vi "pm1-mcu.vi"() -> ()   [LabVIEW 2015]
uses:
  <vilib>/myRIO/Common/Instrument Driver Framework/myRIO v1.0/UART/vis/myRIO v1.0 Close UART.vi
  <vilib>/FPGAPlugInAG/myRIO-1900/niLvFpga_Open_myRIO-1900.vi
  <vilib>/rvi/interface/common/dynamic/niFpgaDynamicAddResources.vi
  <vilib>/imath/engines/lvmath2/RunTimeEngine/BuiltInFunctions/fix/NIMS_fix(DBL-S).vi
  <vilib>/imath/engines/lvmath2/RunTimeEngine/BuiltInFunctions/rand/NIMS_rand().vi
  <vilib>/imath/engines/lvmath2/RunTimeEngine/ErrorHandling/NIMS_Error From Error Code.vi
  <vilib>/imath/engines/lvmath2/RunTimeEngine/NodeEndStatement/NIMS_NodeEndStatement_Output.vi
  <instcachedir>/0/NIMS_NodeEndStatement_Output_53EC0D466D134D7ABD903AC30B43404B.lvgen/NIMS_NodeEndStatement_Output_53EC0D466D134D7ABD903AC30B43404B_010.vi
  <instcachedir>/0/NIMS_NodeEndStatement_Output_53EC0D466D134D7ABD903AC30B43404B.lvgen/NIMS_NodeEndStatement_Output_53EC0D466D134D7ABD903AC30B43404B_001.vi
  <vilib>/imath/engines/lvmath2/RunTimeEngine/ErrorHandling/NIMS_Finalize Error.vi
  <vilib>/Utility/error.llb/Error Cluster From Error Code.vi
  <vilib>/rvi/errors/niLvFpgaAdjustHostInterfaceError.vi
  <vilib>/FPGAPlugInAG/Dynamic/niLvFpga_Close_Dynamic.vi
  <vilib>/myRIO/Common/Instrument Driver Framework/Utilities/vis/FPGA Ref Manager.vi
  <vilib>/myRIO/Common/Instrument Driver Framework/myRIO v1.0/myRIO v1.0 Reset FPGA.vi
  <vilib>/myRIO/Common/Instrument Driver Framework/myRIO v1.0/IRQ/vis/myRIO v1.0 IRQ Info FGV.vi
  <vilib>/myRIO/Common/Instrument Driver Framework/myRIO v1.0/IRQ/vis/myRIO v1.0 Timer IRQ Info FGV.vi
  <vilib>/myRIO/Common/Instrument Driver Framework/myRIO v1.0/IRQ/vis/myRIO v1.0 ISR Agent.vi
  <vilib>/rvi/interface/nirviOpenFPGA/nirviOpenFPGA.xnode
  FPGA Bitfiles/pm1_FPGATarget_pm1-fpga_HhK76n5Wd-Q.lvbitx
  pm1-fpga.vi
  <vilib>/rvi/interface/nirviReadWriteControl/nirviReadWriteControl.xnode
  <vilib>/rvi/interface/nirviCloseFPGA/nirviCloseFPGA.xnode
  <vilib>/myRIO/Instrument Drivers/Utilities/Utilities.lvlib
  NiFpgaLv.dll
  <vilib>/rvi/interface/Simulation/niFpgaSimulationCallBeginRW.vi
panel:
  in  "Time Between Note Change (mSec)":i32
  in  "Test Button Three":bool
  in  "Test Button Two":bool
  in  "Test Button One":bool
  in  "Randomize Inputs for Training Data Input":bool
  out "Number of Buttons Being Pressed":dbl format="%#_13g"
  out "Interval Between Consecutive Notes":dbl format="%#_13g"
  out "Note 6":string
  out "Note 5":string
  out "Note 4":string
  out "Note 3":string
  out "Note 2":string
  out "Note 1":string
  out "Octave6":dbl format="%#_13g"
  out "Octave5":dbl format="%#_13g"
  out "Octave4":dbl format="%#_13g"
  out "Octave3":dbl format="%#_13g"
  out "Octave2":dbl format="%#_13g"
  out "Octave1":dbl format="%#_13g"
  out "Button6":bool
  out "Button5":bool
  out "Button4":bool
  out "Button3":bool
  out "Button2":bool
  out "Button1":bool
  out "Waveform Chart":sgl(graph)
  out "Octave":dbl format="%#_13g"
  out "pitch":dbl format="%#_13g"
  in  "Volume":dbl(slide) scale=0.0..10.0
  out "frequency 6":dbl format="%#_13g"
  out "frequency 5":dbl format="%#_13g"
  out "frequency 4":dbl format="%#_13g"
  out "frequency 3":dbl format="%#_13g"
  out "frequency 2":dbl format="%#_13g"
  out "frequency 1":dbl format="%#_13g"
  out "error out":errorcluster
  in  "stop":bool
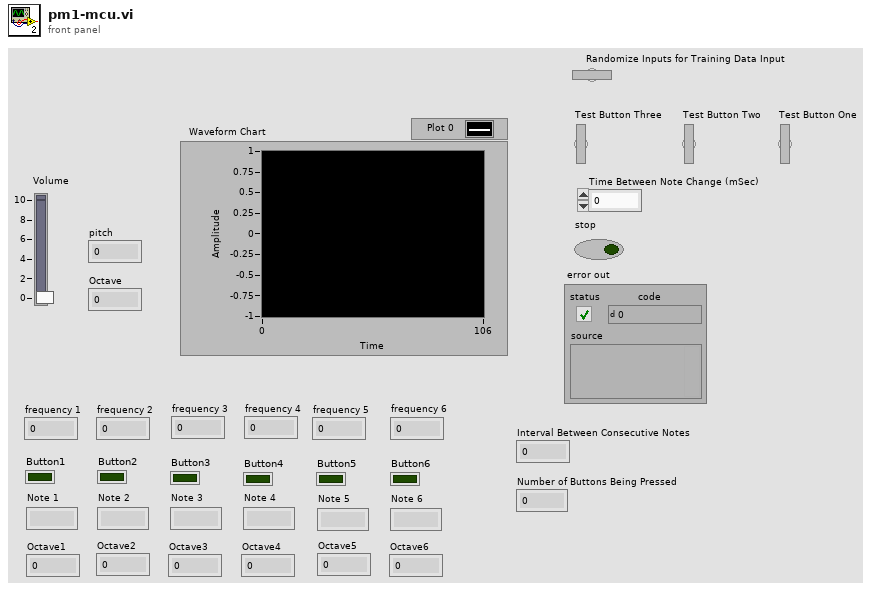
[diagram p1: front panel]
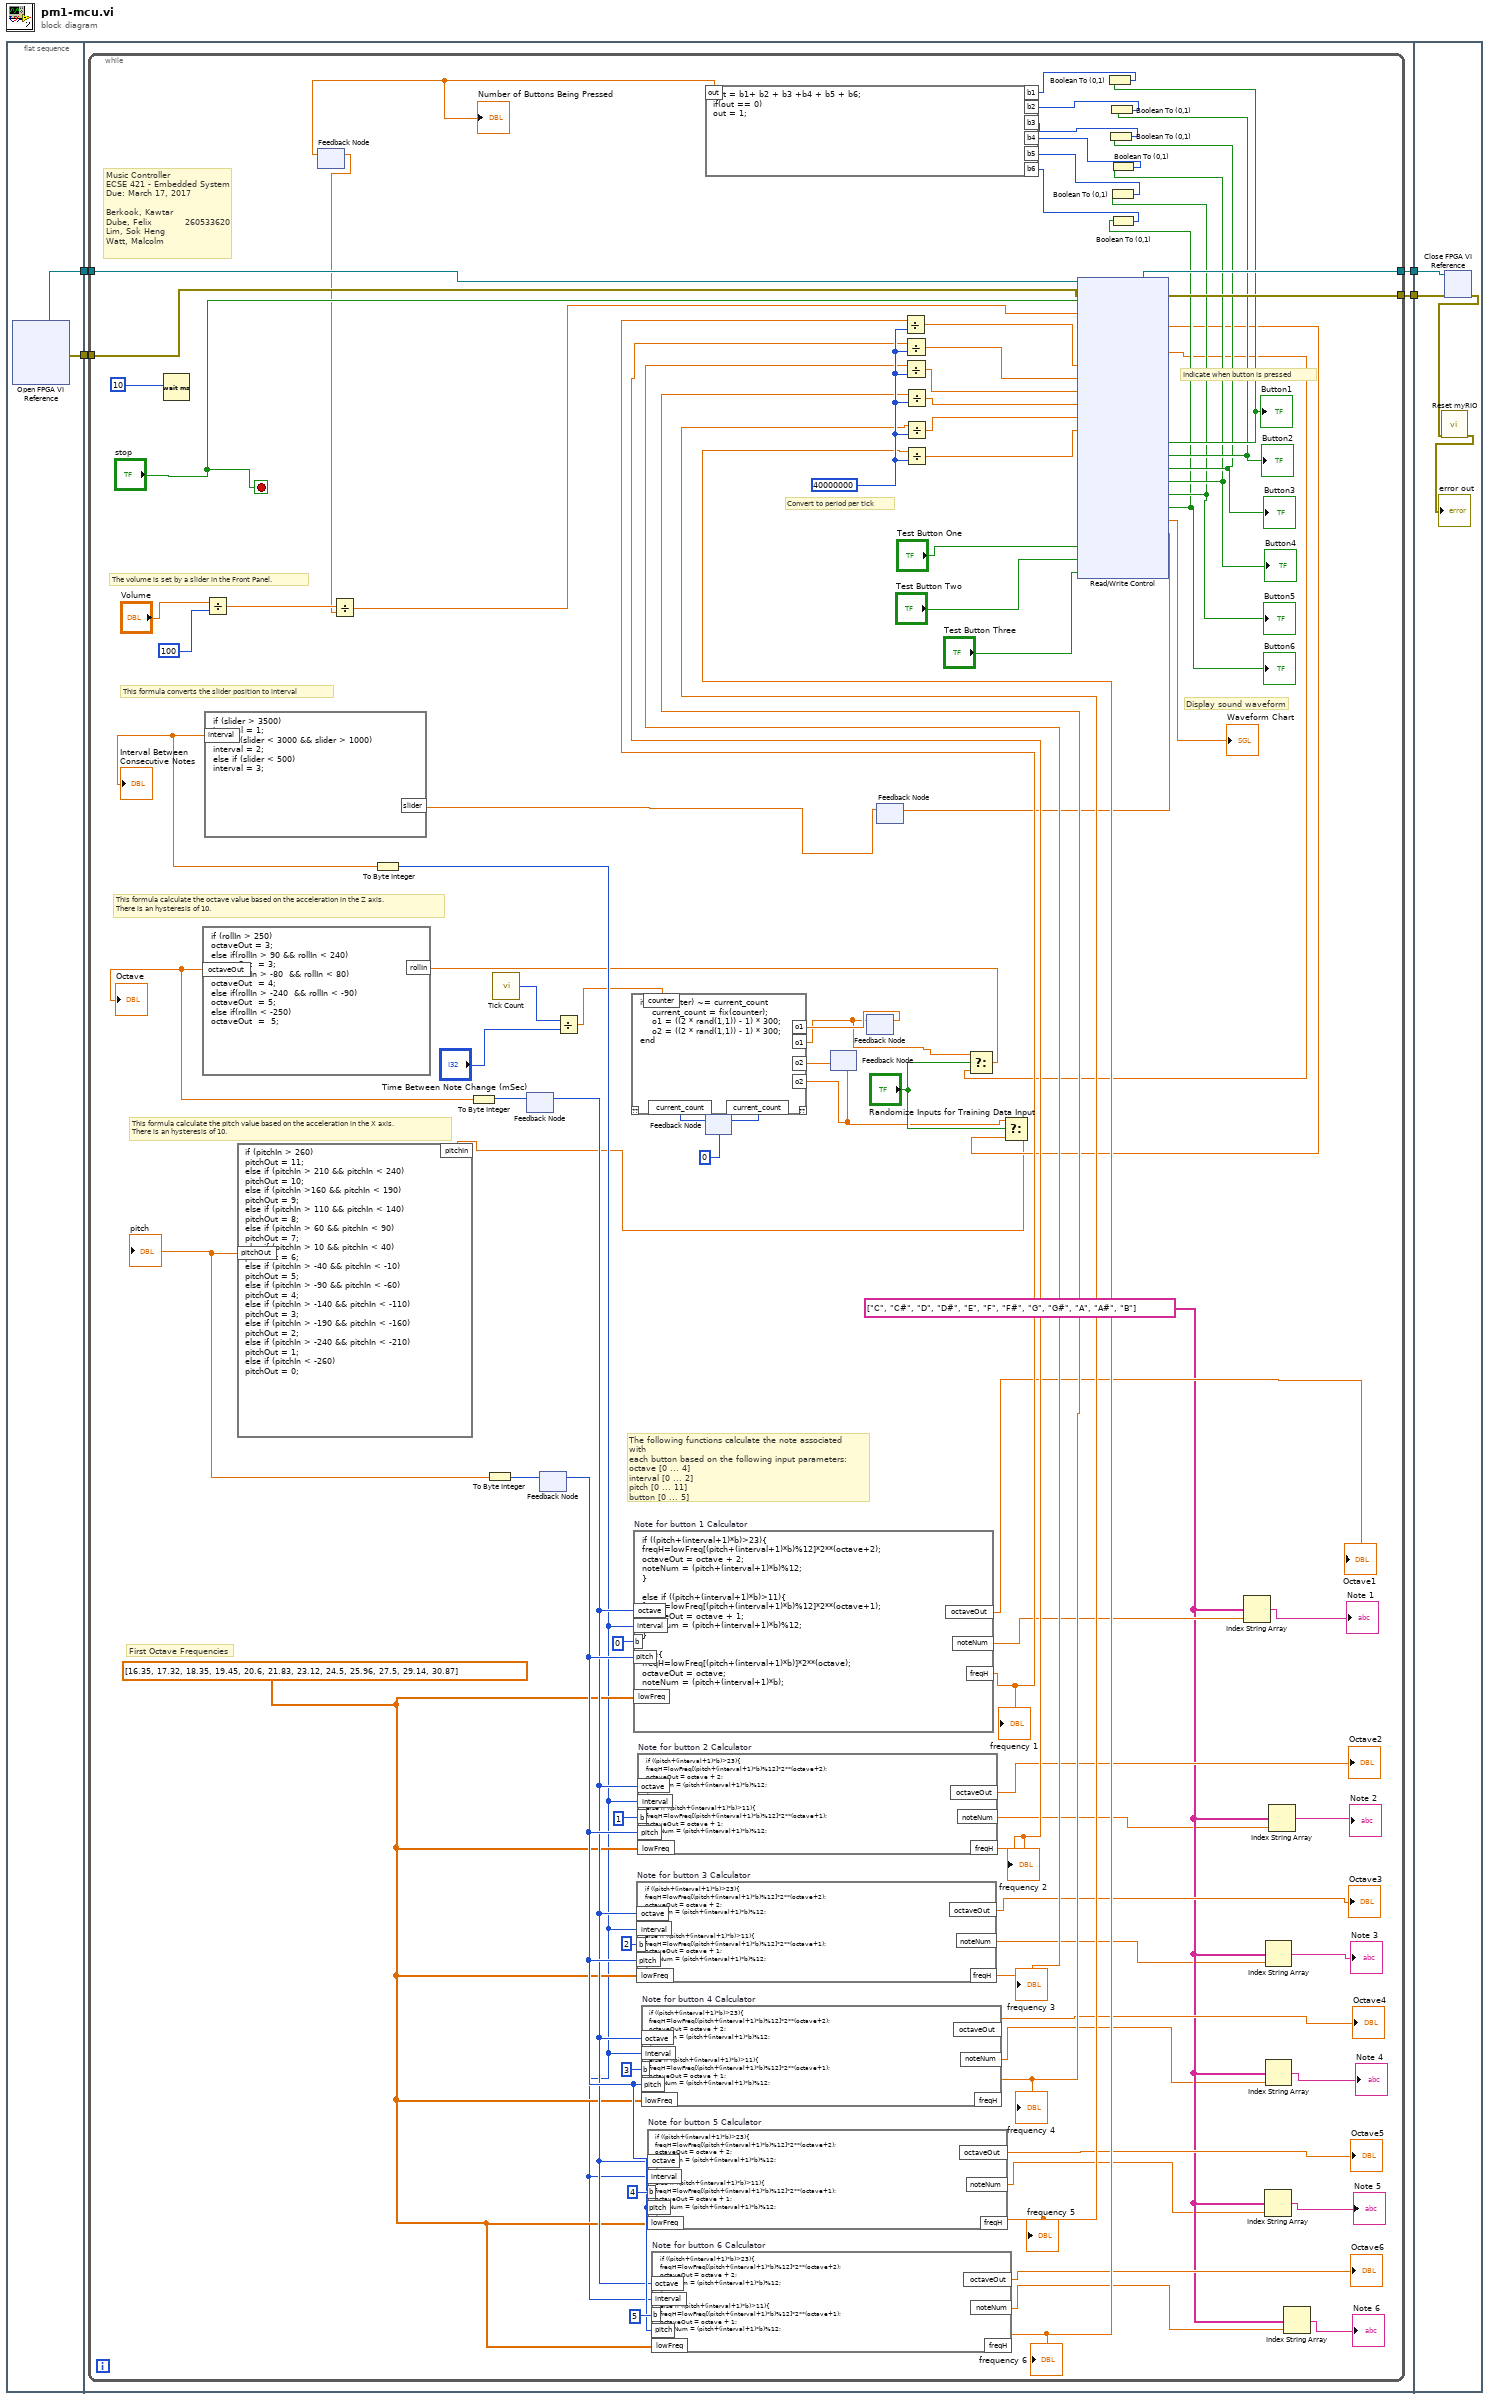
[diagram p0: block diagram]
diagram:
  n1 = flat-sequence {
    tunnel: [w6] -> w4
    tunnel: [w5] -> w2
    tunnel: w4 -> [w10]
    tunnel: [w9] -> w3
    tunnel: w2 -> [w8]
    tunnel: [w7] -> w1
    tunnel: w3 -> [w202]
    tunnel: w1 -> [w201]
    frame #0 {
      n2 = xnode "Open FPGA VI Reference"() -> ("FPGA VI Reference Out"=w6:refnum<k20>, "error out"=w5:errorcluster)  [unwired: 2 in]
    }
    frame #1 {
      n3 = while {
        tunnel: w10 -> [w102]
        tunnel: [w101] -> w9
        tunnel: w8 -> [w99]
        tunnel: [w98] -> w7
        stop <- "stop" stop-if-true
        w60 = string[] ["C", "C#", "D", "D#", "E", "F", "F#", "G", "G#", "A", "A#", "B"]
        w72 = dbl[] [16.35, 17.32, 18.35, 19.45, 20.6, 21.83, 23.12, 24.5, 25.96, 27.5, 29.14, 30.87] ("Low Frequency (Hz) 2")
        w85 = 40000000
        # "This formula converts the slider position to interval"
        # "Music Controller\nECSE 421 - Embedded System\nDue: March 17, 2017\n\nBerkook, Kawtar\nDube, Felix           260533620\nLim, Sok Heng\nWatt, Malcolm"
        # "Convert to period per tick"
        # "Display sound waveform"
        # "Indicate when button is pressed"
        # "The volume is set by a slider in the Front Panel."
        # "This formula calculate the octave value based on the acceleration in the Z axis.\nThere is an hysteresis of 10."
        # "This formula calculate the pitch value based on the acceleration in the X axis.\nThere is an hysteresis of 10."
        # "The following functions calculate the note associated with\neach button based on the following input parameters:\noctave [0 ... 4]\ninterval [0 ... 2]\npitch [0 ... 11]\nbutton [0 ... 5]"
        # "First Octave Frequencies"
        n4 = Wait (ms)(milliseconds to wait=10) -> ()  [unwired: 1 out]
        n5 = Divide(x="Volume", y=100) -> (x/y=w31:dbl)
        n6 = feedback #1() -> (w30:dbl)  [unwired: 1 in]
        n7 = Divide(x=w31, y=w30) -> (x/y=w33:dbl)
        n8 = call "Tick Count"() -> ("Tick Count(mSec)"=w24:u32)
        n9 = feedback #2() -> (w73:i8)  [unwired: 1 in]
        n10 = feedback #3() -> (w76:i8)  [unwired: 1 in]
        n11 = Divide(x=w24, y="Time Between Note Change (mSec)") -> (x/y=w20:dbl)
        n12 = feedback #4(0) -> (w18:u32)
        n13 = feedback #5() -> (w13:dbl)  [unwired: 1 in]
        n14 = feedback #6() -> (w16:dbl)  [unwired: 1 in]
        n15 = mathscript code="if fix(counter) ~= current_count\n    current_count = fix(counter);\n    o1 = ((2 * rand(1,1)) - 1) * 300;\n    o2 = ((2 * rand(1,1)) - 1) * 300;\nend"("counter"=w20, "current_count"=w18, "o1"=w16, "o2"=w13) -> ("current_count"=w19:u32, "o1"=w14:dbl, "o2"=w17:dbl)  [unwired: 1 in, 1 out]
        n16 = feedback-in #4(w19) -> ()
        n17 = feedback-in #5(w17) -> ()
        n18 = feedback-in #6(w14) -> ()
        n19 = feedback #7() -> (w29:sgl)  [unwired: 1 in]
        n20 = formula code="if (slider > 3500)\ninterval = 1;\nelse if (slider < 3000 && slider > 1000)\ninterval = 2;\nelse if (slider < 500)\ninterval = 3;"("slider"=w29) -> ("interval"=w47:dbl)
        "Interval Between Consecutive Notes" <- w47
        n21 = To Byte Integer(number=w47) -> (8bit integer=w48:i8)
        n22 = formula code="if ((pitch+(interval+1)*b)>23){\nfreqH=lowFreq[(pitch+(interval+1)*b)%12]*2**(octave+2);\noctaveOut = octave + 2;\nnoteNum = (pitch+(interval+1)*b)%12;\n}\n\nelse if ((pitch+(interval+1)*b)>11){\nfreqH=lowFreq[(pitch+(interval+1)*b)%12]*2**(octave+1);\noctaveOut = octave + 1;\nnoteNum = (pitch+(interval+1)*b)%12;\n}\n\nelse{\nfreqH=lowFreq[(pitch+(interval+1)*b)]*2**(octave);\noctaveOut = octave;\nnoteNum = (pitch+(interval+1)*b);\n}" "Note for button 1 Calculator"("pitch"=w76, "interval"=w48, "octave"=w73, "b"=0, "lowFreq"=w72) -> ("freqH"=w79:dbl, "octaveOut"=→"Octave1":dbl, "noteNum"=w61:dbl)
        "frequency 1" <- w79
        n23 = formula code="if ((pitch+(interval+1)*b)>23){\nfreqH=lowFreq[(pitch+(interval+1)*b)%12]*2**(octave+2);\noctaveOut = octave + 2;\nnoteNum = (pitch+(interval+1)*b)%12;\n}\n\nelse if ((pitch+(interval+1)*b)>11){\nfreqH=lowFreq[(pitch+(interval+1)*b)%12]*2**(octave+1);\noctaveOut = octave + 1;\nnoteNum = (pitch+(interval+1)*b)%12;\n}\n\nelse{\nfreqH=lowFreq[(pitch+(interval+1)*b)]*2**(octave);\noctaveOut = octave;\nnoteNum = (pitch+(interval+1)*b);\n}" "Note for button 3 Calculator"("pitch"=w76, "interval"=w48, "octave"=w73, "b"=2, "lowFreq"=w72) -> ("freqH"=w81:dbl, "octaveOut"=→"Octave3":dbl, "noteNum"=w57:dbl)
        "frequency 3" <- w81
        n24 = formula code="if ((pitch+(interval+1)*b)>23){\nfreqH=lowFreq[(pitch+(interval+1)*b)%12]*2**(octave+2);\noctaveOut = octave + 2;\nnoteNum = (pitch+(interval+1)*b)%12;\n}\n\nelse if ((pitch+(interval+1)*b)>11){\nfreqH=lowFreq[(pitch+(interval+1)*b)%12]*2**(octave+1);\noctaveOut = octave + 1;\nnoteNum = (pitch+(interval+1)*b)%12;\n}\n\nelse{\nfreqH=lowFreq[(pitch+(interval+1)*b)]*2**(octave);\noctaveOut = octave;\nnoteNum = (pitch+(interval+1)*b);\n}" "Note for button 2 Calculator"("pitch"=w76, "interval"=w48, "octave"=w73, "b"=1, "lowFreq"=w72) -> ("freqH"=w80:dbl, "octaveOut"=→"Octave2":dbl, "noteNum"=w59:dbl)
        "frequency 2" <- w80
        n25 = formula code="if ((pitch+(interval+1)*b)>23){\nfreqH=lowFreq[(pitch+(interval+1)*b)%12]*2**(octave+2);\noctaveOut = octave + 2;\nnoteNum = (pitch+(interval+1)*b)%12;\n}\n\nelse if ((pitch+(interval+1)*b)>11){\nfreqH=lowFreq[(pitch+(interval+1)*b)%12]*2**(octave+1);\noctaveOut = octave + 1;\nnoteNum = (pitch+(interval+1)*b)%12;\n}\n\nelse{\nfreqH=lowFreq[(pitch+(interval+1)*b)]*2**(octave);\noctaveOut = octave;\nnoteNum = (pitch+(interval+1)*b);\n}" "Note for button 4 Calculator"("pitch"=w76, "interval"=w48, "octave"=w73, "b"=3, "lowFreq"=w72) -> ("freqH"=w82:dbl, "octaveOut"=→"Octave4":dbl, "noteNum"=w56:dbl)
        "frequency 4" <- w82
        n26 = formula code="if ((pitch+(interval+1)*b)>23){\nfreqH=lowFreq[(pitch+(interval+1)*b)%12]*2**(octave+2);\noctaveOut = octave + 2;\nnoteNum = (pitch+(interval+1)*b)%12;\n}\n\nelse if ((pitch+(interval+1)*b)>11){\nfreqH=lowFreq[(pitch+(interval+1)*b)%12]*2**(octave+1);\noctaveOut = octave + 1;\nnoteNum = (pitch+(interval+1)*b)%12;\n}\n\nelse{\nfreqH=lowFreq[(pitch+(interval+1)*b)]*2**(octave);\noctaveOut = octave;\nnoteNum = (pitch+(interval+1)*b);\n}" "Note for button 5 Calculator"("pitch"=w76, "interval"=w48, "octave"=w73, "b"=4, "lowFreq"=w72) -> ("freqH"=w83:dbl, "octaveOut"=→"Octave5":dbl, "noteNum"=w54:dbl)
        "frequency 5" <- w83
        n27 = formula code="if ((pitch+(interval+1)*b)>23){\nfreqH=lowFreq[(pitch+(interval+1)*b)%12]*2**(octave+2);\noctaveOut = octave + 2;\nnoteNum = (pitch+(interval+1)*b)%12;\n}\n\nelse if ((pitch+(interval+1)*b)>11){\nfreqH=lowFreq[(pitch+(interval+1)*b)%12]*2**(octave+1);\noctaveOut = octave + 1;\nnoteNum = (pitch+(interval+1)*b)%12;\n}\n\nelse{\nfreqH=lowFreq[(pitch+(interval+1)*b)]*2**(octave);\noctaveOut = octave;\nnoteNum = (pitch+(interval+1)*b);\n}" "Note for button 6 Calculator"("pitch"=w76, "interval"=w48, "octave"=w73, "b"=5, "lowFreq"=w72) -> ("freqH"=w84:dbl, "octaveOut"=→"Octave6":dbl, "noteNum"=w52:dbl)
        "frequency 6" <- w84
        n28 = Divide(x=w79, y=w85) -> (x/y=w91:dbl)
        n29 = Divide(x=w80, y=w85) -> (x/y=w90:dbl)
        n30 = Divide(x=w81, y=w85) -> (x/y=w89:dbl)
        n31 = Divide(x=w82, y=w85) -> (x/y=w88:dbl)
        n32 = Divide(x=w83, y=w85) -> (x/y=w86:dbl)
        n33 = Divide(x=w84, y=w85) -> (x/y=w87:dbl)
        n34 = xnode ("Read/Write Control")("FPGA VI Reference In"=w102, "error in"=w99, "stop"="stop", "volume"=w33, "f1 (periods/tick)"=w91, "f2 (periods/tick)"=w90, "f3 (periods/tick)"=w89, "f4 (periods/tick)"=w88, "f5 (periods/tick)"=w86, "f6 (periods/tick)"=w87, "Test Button One"="Test Button One", "Test Button Two"="Test Button Two", "Test Button Three"="Test Button Three") -> ("FPGA VI Reference Out"=w101:refnum<k20>, "error out"=w98:errorcluster, "AccX"=w25:sgl, "AccZ"=w27:sgl, "b 1"=w45:bool, "b 2"=w43:bool, "b 3"=w41:bool, "b 4"=w39:bool, "b 5"=w37:bool, "b 6"=w35:bool, "Waveform Chart"=→"Waveform Chart":sgl, "slider"=w46:sgl)  [unwired: 1 out]
        "Button1" <- w45
        "Button2" <- w43
        "Button3" <- w41
        "Button4" <- w39
        "Button5" <- w37
        "Button6" <- w35
        n35 = feedback-in #7(w46) -> ()
        n36 = Select(t=w14, s="Randomize Inputs for Training Data Input", f=w27) -> (s? t:f=w28:dbl)
        n37 = formula code="if (rollIn > 250)\noctaveOut = 3;\nelse if(rollIn > 90 && rollIn < 240)\noctaveOut  = 3;\nelse if(rollIn > -80  && rollIn < 80)\noctaveOut  = 4;\nelse if(rollIn > -240  && rollIn < -90)\noctaveOut  = 5;\nelse if(rollIn < -250)\noctaveOut  =  5;"("rollIn"=w28) -> ("octaveOut"=w70:dbl)
        "Octave" <- w70
        n38 = To Byte Integer(number=w70) -> (8bit integer=w74:i8)
        n39 = feedback-in #2(w74) -> ()
        n40 = Select(t=w13, s="Randomize Inputs for Training Data Input", f=w25) -> (s? t:f=w23:dbl)
        n41 = formula code="if (pitchIn > 260)\npitchOut = 11;\nelse if (pitchIn > 210 && pitchIn < 240)\npitchOut = 10;\nelse if (pitchIn >160 && pitchIn < 190)\npitchOut = 9;\nelse if (pitchIn > 110 && pitchIn < 140)\npitchOut = 8;\nelse if (pitchIn > 60 && pitchIn < 90)\npitchOut = 7;\nelse if (pitchIn > 10 && pitchIn < 40)\npitchOut = 6;\nelse if (pitchIn > -40 && pitchIn < -10)\npitchOut = 5;\nelse if (pitchIn > -90 && pitchIn < -60)\npitchOut = 4;\nelse if (pitchIn > -140 && pitchIn < -110)\npitchOut = 3;\nelse if (pitchIn > -190 && pitchIn < -160)\npitchOut = 2;\nelse if (pitchIn > -240 && pitchIn < -210)\npitchOut = 1;\nelse if (pitchIn < -260)\npitchOut = 0;"("pitchIn"=w23) -> ("pitchOut"=w71:dbl)
        "pitch" <- w71
        n42 = To Byte Integer(number=w71) -> (8bit integer=w75:i8)
        n43 = feedback-in #3(w75) -> ()
        n44 = Boolean To (0,1)(Boolean=w45) -> (0, 1=w44:i16)
        n45 = Boolean To (0,1)(Boolean=w41) -> (0, 1=w40:i16)
        n46 = Boolean To (0,1)(Boolean=w43) -> (0, 1=w42:i16)
        n47 = Boolean To (0,1)(Boolean=w37) -> (0, 1=w36:i16)
        n48 = Boolean To (0,1)(Boolean=w39) -> (0, 1=w38:i16)
        n49 = Boolean To (0,1)(Boolean=w35) -> (0, 1=w34:i16)
        n50 = formula code="out = b1+ b2 + b3 +b4 + b5 + b6;\nif(out == 0)\nout = 1;"("b1"=w44, "b2"=w42, "b3"=w40, "b4"=w38, "b5"=w36, "b6"=w34) -> ("out"=w32:dbl)
        "Number of Buttons Being Pressed" <- w32
        n51 = feedback-in #1(w32) -> ()
        n52 = Index String Array(1:w61, 2:w60) -> (0:→"Note 1":string)  [unwired: 1 in]
        n53 = Index String Array(1:w54, 2:w60) -> (0:→"Note 5":string)  [unwired: 1 in]
        n54 = Index String Array(1:w57, 2:w60) -> (0:→"Note 3":string)  [unwired: 1 in]
        n55 = Index String Array(1:w56, 2:w60) -> (0:→"Note 4":string)  [unwired: 1 in]
        n56 = Index String Array(1:w59, 2:w60) -> (0:→"Note 2":string)  [unwired: 1 in]
        n57 = Index String Array(1:w52, 2:w60) -> (0:→"Note 6":string)  [unwired: 1 in]
      }
    }
    frame #2 {
      n58 = xnode "Close FPGA VI Reference"("FPGA VI Reference In"=w202, "error in"=w201) -> ("error out"=w200:errorcluster)
      n59 = call <vilib>:"Reset myRIO.vi"("error in (no error)"=w200) -> ("error out"=→"error out":errorcluster)  [unwired: 10 in]
    }
  }
